vi "Close Device.vi"(8 "error in (no error)":errorcluster, 11 "niDigital in":refnum<class "niDigital.lvclass">) -> (0 "error out":errorcluster, 3 "niDigital out":refnum<class "niDigital.lvclass">)   [LabVIEW 2020, in "niDigital.lvclass"]
uses:
  niDigital.lvclass
  <instrlib>/niDigital/niDigital.llb/niDigital Selected Function.ctl
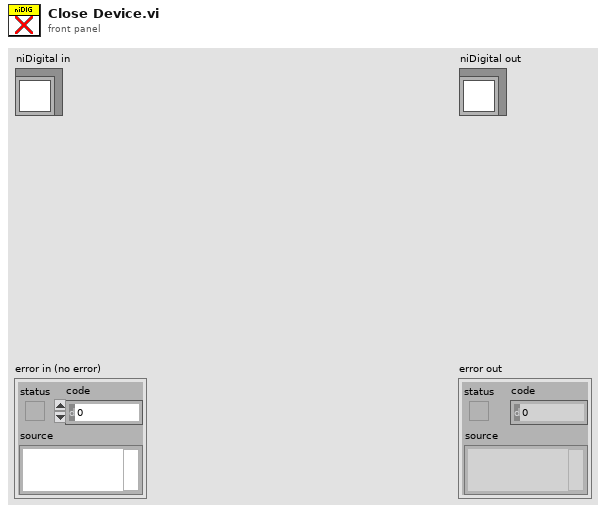
[diagram p1: front panel]
types:
  T1 = typedef "niDigital Selected Function.ctl" = i32
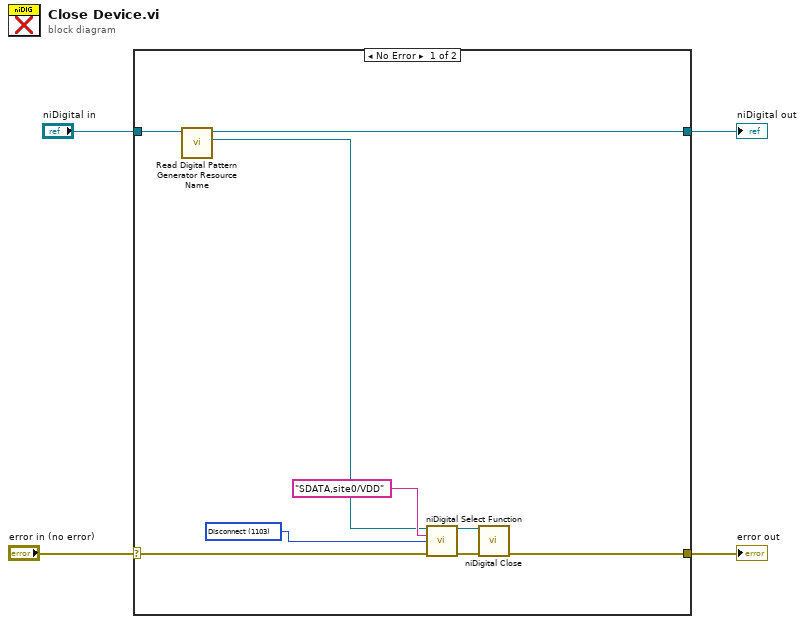
[diagram p0: block diagram]
diagram:
  n1 = case shown="No Error" "error in (no error)" {
    selector: "error in (no error)" -> [w7 w15]
    tunnel: "niDigital in" -> [w13 w14]
    tunnel: [w12 w14] -> w3
    tunnel: [w6 w15] -> w1
    frame No Error {
      w9 = T1 1103 items=["Digital"=1100, "PPMU"=1101, "Off"=1102, "Disconnect"=1103] ("function")
      n2 = call-dynamic "Read Digital Pattern Generator Resource Name.vi"("niDigital in"=w13) -> ("Digital Pattern Generator Resource Name"=w5:refnum<k15>, "niDigital out"=w12:refnum<class "niDigital.lvclass">)  [unwired: 9 in]
      n3 = call <instrlib>:"niDigital Select Function.vi"("instrument handle"=w5, "channel list"="SDATA,site0/VDD" ("Serial Channel List"), "function"=w9, "error in"=w7) -> ("instrument handle out"=w11:refnum<k15>, "error out"=w10:errorcluster)  [unwired: 10 in]
      n4 = call <instrlib>:"niDigital Close.vi"("instrument handle"=w11, "error in"=w10) -> ("error out"=w6:errorcluster)  [unwired: 13 in]
    }
    frame Error {
    }
  }
  "error out" <- w1
  "niDigital out" <- w3
